vi "Actor.vi"(11 "Class":refnum<class "DAQmx - Analog Input Multi Sample.lvclass">) -> ()   [LabVIEW 2021, in "DAQmx - Analog Input Multi Sample.lvclass"]
uses:
  DAQmx - Analog Input Multi Sample.lvclass
  C:/TSA/DAQmx-Bus/Source/DAQmx-Bus.lvclass
  DAQmx-Bus.lvclass/DAQmx-Bus.ctl
  DAQmx - Analog Input Multi Sample.lvclass/DAQmx - Analog Input Multi Sample.ctl
  <vilib>/Platform/TimedLoop/XDataNode/timing_clust.ctl
  <vilib>/Platform/TimedLoop/XDataNode/nitl_modes.ctl
  <vilib>/Platform/TimedLoop/XDataNode/wakeup.ctl
  <vilib>/DAQmx/read.llb/DAQmx Read (Analog 1D Wfm NChan NSamp).vi
  Properties/Read DAQmx Task.vi
  Properties/Read Update Rate.vi
  Properties/Read timeout.vi
  Properties/Read Values DVR.vi
  Properties/Read Stop.vi
  Properties/Read Sync.vi
  <vilib>/DAQmx/miscellaneous.llb/DAQmx Fill In Error Info.vi
  <vilib>/platform/TimedLoop/XDataNode/XDataNode.xnode
  <resource>/objmgr/daqmx.rc
  <vilib>/Platform/TimedLoop/XDataNode/XDNodeRunTimeDep.lvlib
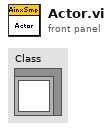
[diagram p1: front panel]
types:
  T1 = typedef "XDNodeRunTimeDep.lvlib/timing_clust.ctl" = cluster{"Expected End [f-1]":u64, "Actual End [f-1]":u64, "Finished Late? [f-1]":bool, "Expected End [i-1]":u64, "Actual End [i-1]":u64, "Finished Late? [i-1]":bool, "Expected Start [i]":u64, "Actual Start [i]":u64, "Expected Start [f]":u64, "Actual Start [f]":u64, "Source Name":string, "Structure Name":string, "Period":i64, "Deadline":i64, "Offset":i64, "Start":i64, "Priority":i32, "Timeout":i32, "Mode":T2, "Wakeup Reason":T3, "Error":errorcluster, "Source Type":string, "Secondary Source Type":string, "Global End Time":u64, "Global Start Time":u64, "Frame Duration":u64, "Iteration Duration":u64, "Assigned CPU":i32, "I/O Scan Engine Mode":u32}
  T2 = typedef "XDNodeRunTimeDep.lvlib/nitl_modes.ctl" = enum32{"No Change", "Process missed periods, maintain original phase", "Discard missed periods, maintain original phase", "Process missed periods, ignore original phase", "Discard missed periods, ignore original phase"}
  T3 = typedef "XDNodeRunTimeDep.lvlib/wakeup.ctl" = enum32{"Normal", "Aborted", "Asynchronous wakeup", "Timing source error", "Timed loop error", "Timeout"}
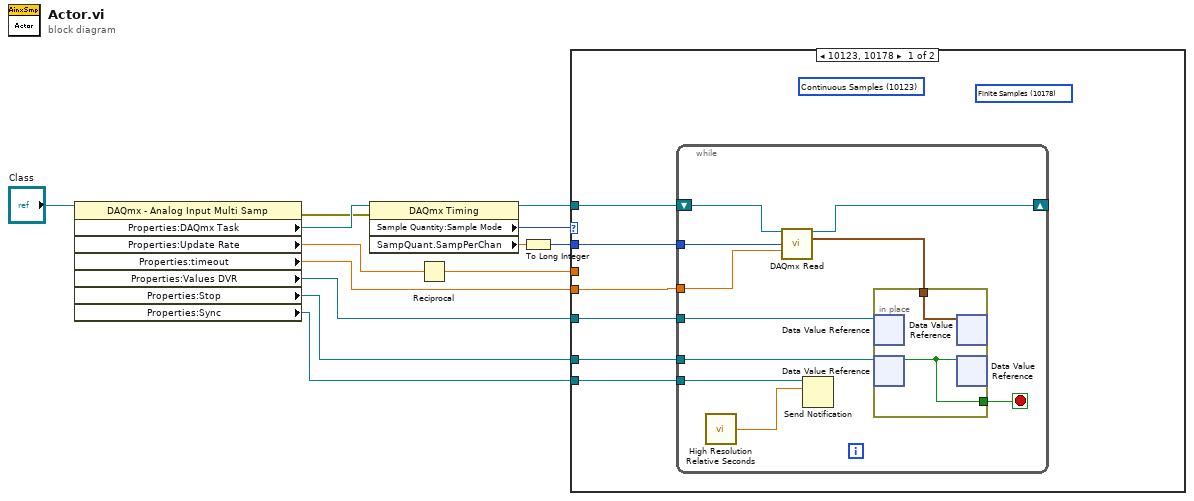
[diagram p0: block diagram]
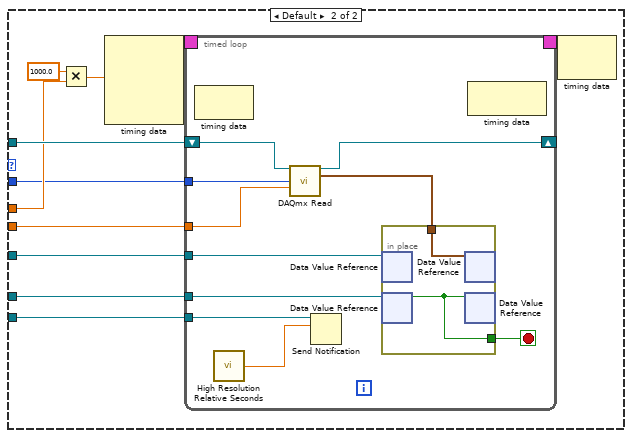
[diagram p2: hidden frame]
diagram:
  n1 = property class="DAQmx - Analog Input Multi Samp"(reference="Class") -> (error out=w8:errorcluster, "Properties:DAQmx Task"=w9:refnum<k21>, "Properties:Update Rate"=w5:dbl, "Properties:timeout"=w12:dbl, "Properties:Values DVR"=w11:refnum<data-value>, "Properties:Stop"=w13:refnum<data-value>, "Properties:Sync"=w10:refnum<notifier>)  [unwired: 1 in, 1 out]
  n2 = property class="DAQmx Timing"(reference=w9, error in=w8) -> (reference out=w7:refnum<k21>, "Sample Quantity:Sample Mode"=w6:i32, "SampQuant.SampPerChan"=w2:dbl)  [unwired: 1 out]
  n3 = Reciprocal(x=w5) -> (1/x=w4:dbl)
  n4 = To Long Integer(number=w2) -> (32bit integer=w1:i32)
  n5 = case shown="10123, 10178" w6 {
    tunnel: w13 -> [w19 w42]
    tunnel: w12 -> [w15 w41]
    tunnel: w11 -> [w18 w40]
    tunnel: w10 -> [w17 w39]
    tunnel: w7 -> [w16 w38]
    tunnel: w4 -> [_ w35]
    tunnel: w1 -> [w14 w32]
    frame 10123, 10178 {
      (unwired) 10178 items=["Finite Samples"=10178, "Continuous Samples"=10123, "Hardware Timed Single Point"=12522] ("SampQuant.SampMode")
      (unwired) 10123 items=["Finite Samples"=10178, "Continuous Samples"=10123, "Hardware Timed Single Point"=12522] ("SampQuant.SampMode")
      n6 = while {
        shift-right: [w28] -> _
        shift-left: w16 -> [w29]
        tunnel: w19 -> [w27]
        tunnel: w15 -> [w25]
        tunnel: w18 -> [w24]
        tunnel: w17 -> [w21]
        tunnel: w14 -> [w20]
        stop <- w26 stop-if-true
        n7 = call <vilib>:"High Resolution Relative Seconds.vi"() -> ("relative seconds"=w22:dbl)
        n8 = call-poly <vilib>:"DAQmx Read.vi"("task/channels in"=w29, "number of samples per channel"=w20, "timeout"=w25) -> ("task out"=w28:refnum<k21>, "data"=w23:waveform(dbl)[])  [unwired: 10 in, 1 out]
        n9 = Send Notification(notification=w22, notifier=w21) -> ()  [unwired: 1 in, 2 out]
        n10 = in-place {
          in-place-border: [w31] -> w26
          in-place-border: w23 -> [w30]
          n11 = in-place-dvr #1(w24) -> ()  [unwired: 2 out]
          n12 = in-place-dvr #2(w27) -> (w31:bool)  [unwired: 1 out]
          n13 = in-place-dvr #1(w30) -> ()  [unwired: 2 out]
          n14 = in-place-dvr #2(w31) -> ()  [unwired: 2 out]
        }
      }
    }
    frame Default {
      n15 = Multiply(x=1000.0, y=w35) -> (x*y=w33:dbl)
      n16 = node-c288(w33) -> (w37:T1)  [unwired: 3 in]
      n17 = timed-loop {
        shift-right: [w51] -> _
        shift-left: w38 -> [w52]
        tunnel: w42 -> [w50]
        tunnel: w41 -> [w48]
        tunnel: w40 -> [w47]
        tunnel: w39 -> [w44]
        timing: w37 -> [_]
        timing-out: [_] -> w36
        tunnel: w32 -> [w43]
        stop <- w49 stop-if-true
        n18 = node-c288() -> ()  [unwired: 1 in, 1 out]
        n19 = call <vilib>:"High Resolution Relative Seconds.vi"() -> ("relative seconds"=w45:dbl)
        n20 = call-poly <vilib>:"DAQmx Read.vi"("task/channels in"=w52, "number of samples per channel"=w43, "timeout"=w48) -> ("task out"=w51:refnum<k21>, "data"=w46:waveform(dbl)[])  [unwired: 10 in, 1 out]
        n21 = Send Notification(notification=w45, notifier=w44) -> ()  [unwired: 1 in, 2 out]
        n22 = in-place {
          in-place-border: [w56] -> w49
          in-place-border: w46 -> [w55]
          n23 = in-place-dvr #3(w47) -> ()  [unwired: 2 out]
          n24 = in-place-dvr #4(w50) -> (w56:bool)  [unwired: 1 out]
          n25 = in-place-dvr #3(w55) -> ()  [unwired: 2 out]
          n26 = in-place-dvr #4(w56) -> ()  [unwired: 2 out]
        }
        n27 = node-c288() -> ()  [unwired: 1 in, 1 out]
      }
      n28 = node-c288(w36) -> ()  [unwired: 1 out]
    }
  }
